vi "globals_9.vi"() -> ()   [LabVIEW 2013]
panel:
  in  "counter_data":dbl
  in  "counter_mode":string
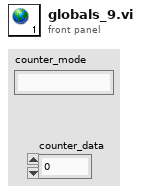
[diagram p1: front panel]
diagram:
